vi "Close OOB.vi"(8 "error in":errorcluster, 11 "OOB in":refnum<class "CIFOutOfBand.lvclass">) -> (0 "error out":errorcluster)   [LabVIEW 2021, in "CIFOutOfBand.lvclass"]
uses:
  CIFOutOfBand.lvclass
  CIFOutOfBand.lvclass/CIFOutOfBand.ctl
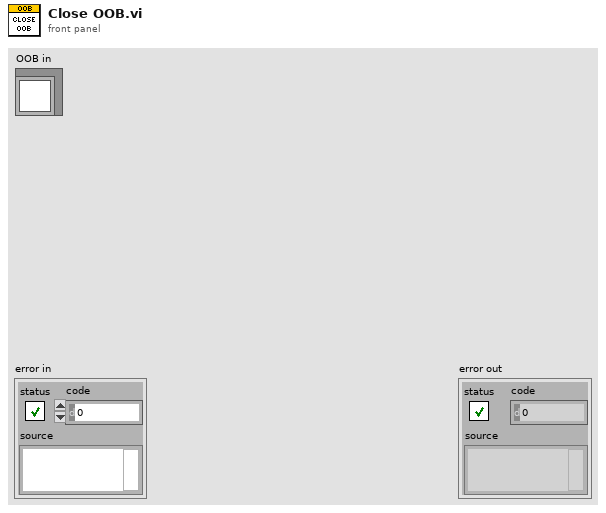
[diagram p1: front panel]
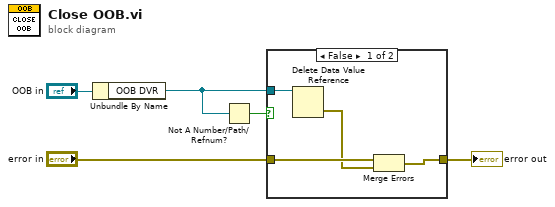
[diagram p0: block diagram]
diagram:
  n1 = Unbundle By Name("OOB in") -> ("OOB DVR"=w3:refnum<data-value>)
  n2 = Not A Number/Path/Refnum?(number/path/refnum=w3) -> (NaN/Path/Refnum?=w5:bool)
  n3 = case shown="False" w5 {
    tunnel: "error in" -> [w9 w10]
    tunnel: [w7 w10] -> w1
    tunnel: w3 -> [w6 _]
    frame False {
      n4 = Delete Data Value Reference(data value reference=w6) -> (error out=w8:errorcluster)  [unwired: 1 in, 1 out]
      n5 = Merge Errors(w9, w8) -> (w7:errorcluster)
    }
    frame True {
    }
  }
  "error out" <- w1
